vi "Load Config.vi"(6 "Constants":refnum<class "Sequence Constants.lvclass">, 8 "error in (no error)":refnum<class "MultiErrors.lvclass">, 10 "Config Element":refnum<class "Config Element.lvclass">, 11 "Save Var Command Config in":refnum<class "Save Var Command Config.lvclass">) -> (0 "error out":refnum<class "MultiErrors.lvclass">, 3 "Save Var Command Config out":refnum<class "Save Var Command Config.lvclass">)   [LabVIEW 2020, in "VolatusSeqConfig.lvlib" / "Save Var Command Config.lvclass"]
uses:
  Save Var Command Config.lvclass
  Save Var Command Config.lvclass/Save Var Command Config.ctl
  lv-cdm/CDM-Config/Config Element/Config Element.lvclass
  VolatusErrorUtilities/MultiErrors/MultiErrors.lvclass
  Sequence Constants/Sequence Constants.lvclass
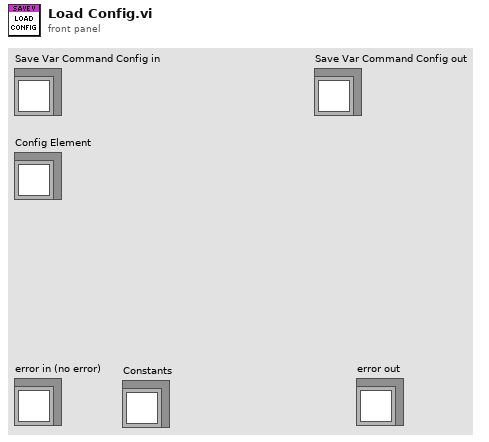
[diagram p1: front panel]
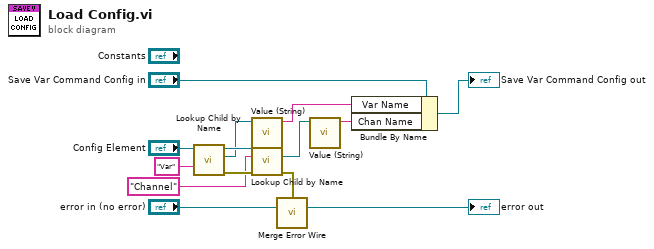
[diagram p0: block diagram]
diagram:
  n1 = call "Lookup Child by Name.vi"("Name"="Var", "Config Element in"="Config Element") -> ("error out"=w14:errorcluster, "Child"=w8:refnum<class "Config Element.lvclass">, "Config Element out"=w10:refnum<class "Config Element.lvclass">)  [unwired: 6 in, 1 out]
  n2 = call "Value (String).vi"("Config Element in"=w8) -> ("String Value"=w4:string)  [unwired: 9 in, 1 out]
  n3 = call "Lookup Child by Name.vi"("error in (no error)"=w14, "Name"="Channel", "Config Element in"=w10) -> ("error out"=w1:errorcluster, "Child"=w7:refnum<class "Config Element.lvclass">)  [unwired: 5 in, 2 out]
  n4 = call "Merge Error Wire.vi"("error in (no error)"=w1, "MultiErrors in"="error in (no error)") -> ("MultiErrors out"=→"error out":refnum<class "MultiErrors.lvclass">)  [unwired: 13 in]
  n5 = call "Value (String).vi"("Config Element in"=w7) -> ("String Value"=w5:string)  [unwired: 9 in, 1 out]
  n6 = Bundle By Name(cluster="Save Var Command Config in", "Var Name"=w4, "Chan Name"=w5) -> (→"Save Var Command Config out":refnum<class "Save Var Command Config.lvclass">)
